vi "Run_JumboBooks.vi"   [LabVIEW 2014]
panel:
  # "Launching JumboBooks"
types:
  T1 = enum32{"Invalid", "Standard", "Closed", "Hidden", "Minimized", "Maximized"}
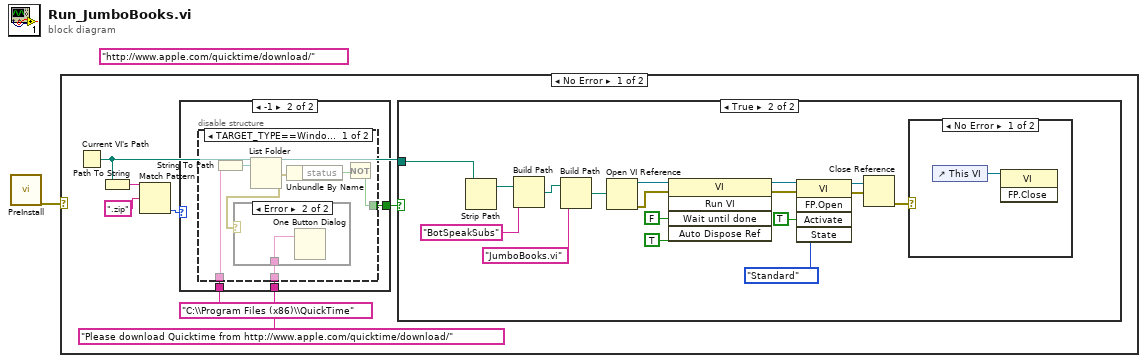
[diagram p0: block diagram]
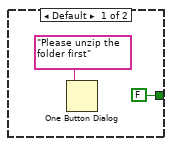
[diagram p4: hidden frame]
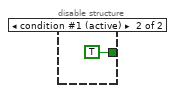
[diagram p6: hidden frame]
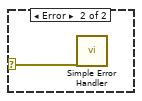
[diagram p7: hidden frame]
diagram:
  (unwired) "http://www.apple.com/quicktime/download/" ("regular expression")
  n1 = call "PreInstall.vi"() -> ("error out"=w1:errorcluster)  [unwired: 3 in]
  n2 = case shown="No Error" w1 {
    selector: w1 -> [_ w40]
    frame No Error {
      n3 = Current VI's Path() -> (path=w4:path)
      n4 = Path To String(path=w4) -> (string=w8:string)
      n5 = Match Pattern(string=w8, regular expression=".zip") -> (offset past match=w6:i32)  [unwired: 1 in, 3 out]
      n6 = case shown="-1" w6 {
        tunnel: [FALSE w31] -> w5
        tunnel: "C:\\Program Files (x86)\\QuickTime" ("regular expression") -> [_ w30]
        tunnel: "Please download Quicktime from http://www.apple.com/quicktime/download/" ("message") -> [_ w29]
        frame Default {
          n7 = One Button Dialog(message="Please unzip the folder first") -> ()  [unwired: 1 in, 1 out]
        }
        frame -1 {
          n8 = disable-structure shown="TARGET_TYPE==Windows" {
            disable-tunnel: [w37 TRUE] -> w31
            disable-tunnel: w30 -> [w36 _]
            disable-tunnel: w29 -> [w35 _]
            frame condition #0 {
              n9 = String To Path(string=w36) -> (path=w34:path)
              n10 = List Folder(path=w34) -> (error out=w32:errorcluster)  [unwired: 3 in, 3 out]
              n11 = case shown="Error" w32 {
                tunnel: w35 -> [_ w38]
                frame No Error {
                }
                frame Error {
                  n12 = One Button Dialog(message=w38) -> ()  [unwired: 1 in, 1 out]
                }
              }
              n13 = Unbundle By Name(w32) -> ("status"=w33:bool)
              n14 = Not(x=w33) -> (.not. x?=w37:bool)
            }
            frame condition #1 (active) {
            }
          }
        }
      }
      n15 = case shown="True" w5 {
        tunnel: w4 -> [_ w9]
        frame False {
        }
        frame True {
          n16 = Strip Path(path=w9) -> (stripped path=w25:path)  [unwired: 1 out]
          n17 = Build Path(base path=w25, name or relative path="BotSpeakSubs") -> (appended path=w24:path)
          n18 = Build Path(base path=w24, name or relative path="JumboBooks.vi") -> (appended path=w21:path)
          n19 = Open VI Reference(vi path=w21) -> (vi reference=w20:refnum<vi>, error out=w19:errorcluster)  [unwired: 5 in]
          n20 = invoke class="VI" method="Run VI"(reference=w20, error in=w19, "Wait until done"=FALSE ("Wait Until Done"), "Auto Dispose Ref"=TRUE ("Auto Dispose Reference")) -> (reference out=w15:refnum<vi>, error out=w14:errorcluster)  [unwired: 1 in, 3 out]
          n21 = invoke class="VI" method="FP.Open"(reference=w15, error in=w14, "Activate"=TRUE ("Activate?"), "State"=T1."Standard") -> (reference out=w12:refnum<vi>, error out=w13:errorcluster)  [unwired: 1 in, 3 out]
          n22 = Close Reference(reference=w12, error in (no error)=w13) -> (error out=w16:errorcluster)
          n23 = case shown="No Error" w16 {
            frame No Error {
              n24 = control-ref of="This VI"() -> (w26:refnum<vi>)
              n25 = invoke class="VI" method="FP.Close"(reference=w26) -> ()  [unwired: 2 in, 3 out]
            }
            frame Error {
            }
          }
        }
      }
    }
    frame Error {
      n26 = call <vilib>:"Simple Error Handler.vi"("error in (no error)"=w40) -> ()  [unwired: 4 in, 5 out]
    }
  }
